vi "Manual Shooter Mode.vi"(10 "Manual Shoot":T1) -> (0 "Shooter Ready?":bool, 1 "Trigger Output":dbl, 2 "Right Output":dbl, 3 "Left Output":dbl, 4 "Angle Motor Out":dbl)   [LabVIEW 2015]
uses:
  Common Code/Manual Shoot.ctl
  Robot Global Data.vi
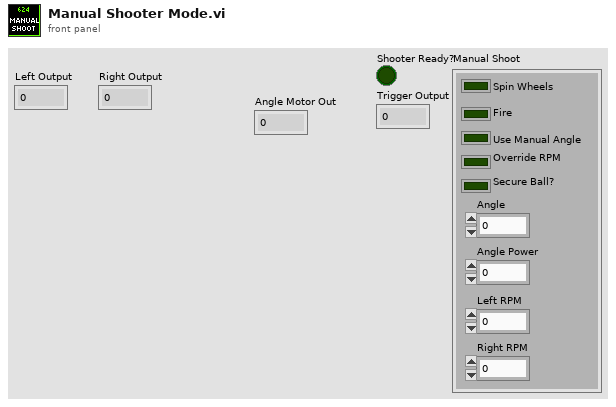
[diagram p1: front panel]
types:
  T1 = typedef "Manual Shoot.ctl" = cluster{"Spin Wheels":bool, "Fire":bool, "Angle":dbl, "Angle Power":dbl, "Use Manual Angle":bool, "Override RPM":bool, "Left RPM":dbl, "Right RPM":dbl, "Secure Ball?":bool}
  T2 = typedef "Dashboard Control Data.ctl" = cluster{"Shooter Presets":T3, "Encoder Control":T5, "Steer PID output":cluster{"output high":dbl, "output low":dbl}, " Steer PID gains":cluster{"proportional gain (Kc)":dbl, "integral time (Ti, min)":dbl, "derivative time (Td, min)":dbl}, "Drivetrain Settings":T6, "Vision Packet":T7, "Dashboard Drivetrain Command":T8, "Info/Command Cluster":T10, "Ball Vision Packet":T11, "Intake Presets":T13, "Intake Encoder Control":T15, "Climb Presets":T16, "Ultrasonic Limit":dbl, "Roll Limit":dbl, "Pitch Limit":dbl, "Goal Output Range":cluster{"output high":dbl, "output low":dbl}}
  T3 = typedef "Shooter Presets.ctl" = cluster{"Batter Shot":T4, "Deep Middle Shot":T4, "Manual Shot":T4, "Left Ticks Per Rotation":dbl, "Right Ticks Per Rotation":dbl, "Low Bar Shot":T4, "Shooter RPM Tolerance":dbl, "IIR Filter Power":dbl, "Trigger Power":dbl, "Fire from Load Delay":i32, "Angle Pot M":dbl, "Angle Pot B":dbl, "Shooter Length":dbl, "String Pot Dist":dbl, "Angle PID gains":cluster{"proportional gain (Kc)":dbl, "integral time (Ti, min)":dbl, "derivative time (Td, min)":dbl}, "Angle Motor Output":cluster{"output high":dbl, "output low":dbl}, "Shooter Angle Tolerance":dbl, "Vision Shoot x^2":dbl, "Vision Shoot x":dbl, "Dist from Axis Cam to Pivot":dbl, "High Goal Center Height":dbl, "Feed Forward Max Accel":dbl, "Feed Forward Kv":dbl, "Backwards Trigger":dbl, "Shot Finish Delay (ms)":dbl, "Angle Max Current":dbl, "Angle Current Trip Time":dbl, "Shooter Intake Angle":dbl, "Vision Shoot c":dbl, "Reset?":bool, "Servo Release Delay":dbl, "Servo Idle Angle":i32, "Servo Hold Angle":i32, "Angle Pot x^2":dbl, "Angle Pot x":dbl, "Angle Pot c":dbl, "Ignore Angle?":bool}
  T4 = typedef "Shot Presets.ctl" = cluster{"Left Wheel RPM":dbl, "Right Wheel RPM":dbl, "Angle":dbl}
  T5 = typedef "Encoder Control.ctl" = cluster{"Right Tick Constant":dbl, "Left Tick Constant":dbl, "Reset?":bool, "Y Dist":cluster{"PID gains":cluster{"proportional gain (Kc)":dbl, "integral time (Ti, min)":dbl, "derivative time (Td, min)":dbl}}, "Y Stop Thresh":dbl, "Y Stop Speed":dbl}
  T6 = typedef "Drivetrain Settings.ctl" = cluster{"Gyro Tolerance":dbl, "Throttle Ramp (ms)":dbl, "Angular rate compensation":bool, "Throttle to Rate Scale":dbl, "Rate compensation gain":dbl, "Kv":dbl, "Ka":dbl, "Feed Forward P":dbl, "Feed Forward D":dbl, "Goal Vision PID gains":cluster{"proportional gain (Kc)":dbl, "integral time (Ti, min)":dbl, "derivative time (Td, min)":dbl}, "Goal Detection Window":dbl}
  T7 = typedef "Goal Vision Packet.ctl" = cluster{"Distance":dbl, "Center X":dbl, "Center Y":dbl, "Found Target?":bool}
  T8 = typedef "Dashboard Drivetrain Command.ctl" = cluster{"Drivetrain Vision":T9}
  T9 = typedef "Drivetrain Vision.ctl" = cluster{"Goal Window":dbl, "Ball Window":dbl}
  T10 = typedef "Ball Tracking Command Cluster.ctl" = cluster{"Distance to Ball":dbl, "Desired Angle":dbl, "Command":enum16{"Turn to Ball", "Turn to Angle", "Get Distance"}, "Pixels from Center":dbl}
  T11 = typedef "Ball Vision Packet.ctl" = cluster{"Ball Detected?":bool, "Distance to Ball":dbl, "Desired Angle":dbl, "Pixels from Center":dbl, "Tracking mode":T12}
  T12 = typedef "Tracking Mode.ctl" = enum16{"Turn to Ball", "Turn to Angle"}
  T13 = typedef "Intake Presets.ctl" = cluster{"Intake Speed":dbl, "Outake Speed":dbl, "Low Height":dbl, "Half Height":dbl, "Full Height":dbl, "Angle Speed":dbl, "Fast Angle":dbl, "Encoder Scale":dbl, "Load Height":dbl, "Output Range":T14, "Rotation Power Max/Min":dbl, "MaxCurrent":dbl, "Intake Trip Time":dbl, "Idle Height":dbl, "Max Height":dbl, "Reset Encoders?":bool, "PID gains":cluster{"proportional gain (Kc)":dbl, "integral time (Ti, min)":dbl, "derivative time (Td, min)":dbl}}
  T14 = typedef "Drivetrain Output Range.ctl" = cluster{"output high":dbl, "output low":dbl}
  T15 = typedef "IntakeEcoderControl.ctl" = cluster{"Arm Tick Constant":dbl, "Reset?":bool, "Y Dist":cluster{"PID gains":cluster{"proportional gain (Kc)":dbl, "integral time (Ti, min)":dbl, "derivative time (Td, min)":dbl}}, "Y Stop Thresh":dbl, "Y Stop Speed":dbl}
  T16 = typedef "Climb Presets.ctl" = cluster{"Pull Power":dbl, "Unpin Power":dbl, "Time to Hold":dbl}
  T17 = typedef "WPI_MotorControlDeviceRef.ctl" = cluster{"DeviceStatus":errorcluster, "Type":T18, "PWM":cluster{"PWM Channel":T19, "DeadBand":T20}, "CAN":cluster{"Device Number":u8, "Control Mode":T21, "Semaphore":T22, "Max Vout":dbl, "TalonSRX Control Mode":T23}, "Invert":bool}
  T18 = typedef "WPI_MotorControlType.ctl" = enum16{"PWM", "CAN", "CANTalonSRX"}
  T19 = typedef "FPGA_DIOPWMChannel.ctl" = enum8{"PWM 0", "PWM 1", "PWM 2", "PWM 3", "PWM 4", "PWM 5", "PWM 6", "PWM 7", "PWM 8", "PWM 9", "PWM MXP 0", "PWM MXP 1", "PWM MXP 2", "PWM MXP 3", "PWM MXP 4", "PWM MXP 5", "PWM MXP 6", "PWM MXP 7", "PWM MXP 8", "PWM MXP 9", "Invalid"}
  T20 = typedef "WPI_PWMDeadband.ctl" = cluster{"Name":string, "maxPositivePwm":i32, "minPositivePwm":i32, "centerPwm":i32, "maxNegativePwm":i32, "minNegativePwm":i32, "angularRange":u16}
  T21 = typedef "WPI_CANJaguar_ControlMode.ctl" = enum8{"Percent VBus", "Current", "Speed", "Position", "Voltage"}
  T22 = typedef "Semaphore RefNum" = refnum<k1>
  T23 = typedef "WPI_CANTalonSRX_APIControlMode.ctl" = enum8{"Percent VBus", "Speed", "Position", "Slave", "Unchanged / Invalid", "Voltage Compensation", "Current", "Motion Profile"}
  T24 = typedef "Intake Status Cluster.ctl" = cluster{"Roller Power":dbl, "Angle Power":dbl, "Intake Mode":T25, "Intake States":T26, "Rollers Active?":bool, "Current Height":dbl, "Target Height":dbl, "Encoder Raw Position":dbl, "Forward Tripped?":bool, "Backward Tripped?":bool, "Override IR?":bool}
  T25 = typedef "Intake Mode.ctl" = enum16{"Safe", "Auto", "Manual"}
  T26 = typedef "Intake States.ctl" = enum16{"Idle", "Set roller speed", "Move to angle"}
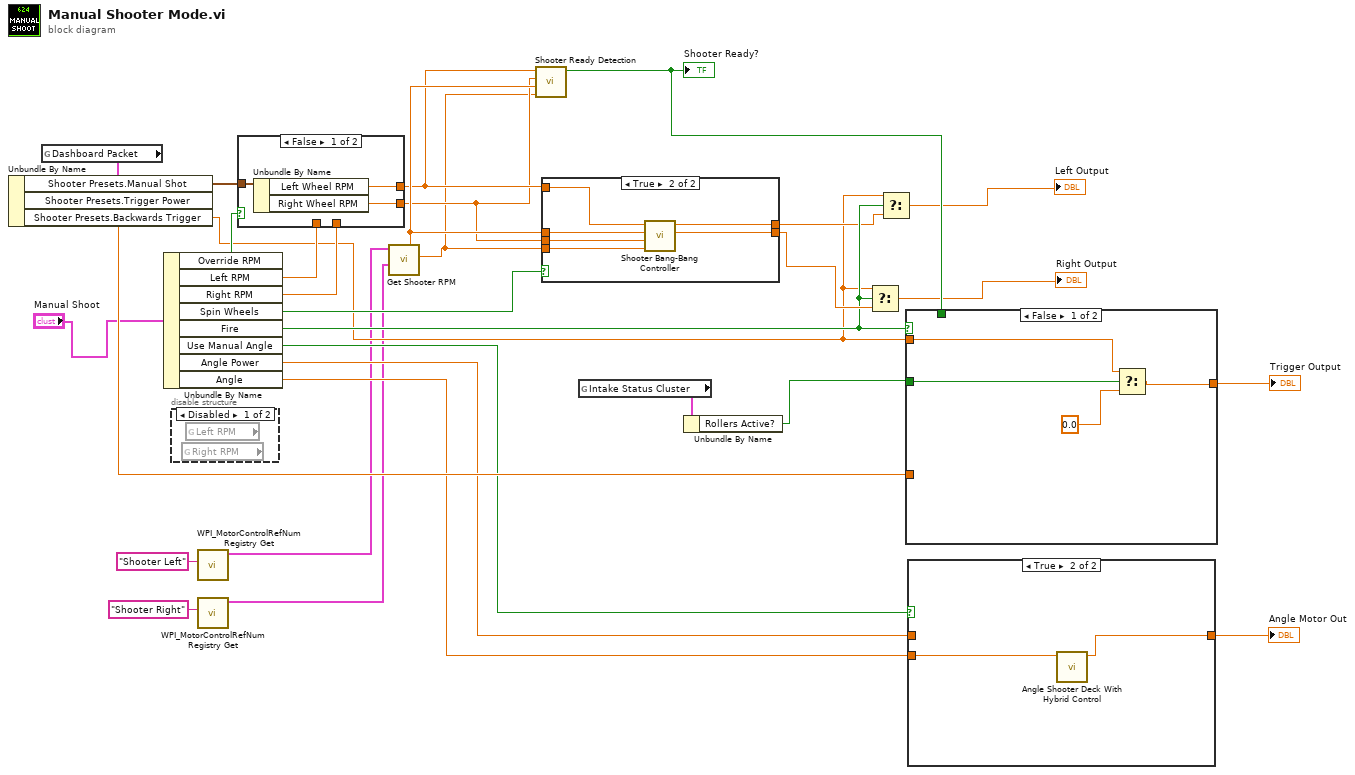
[diagram p0: block diagram]
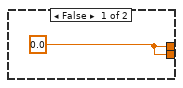
[diagram p6: hidden frame]
diagram:
  n1 = global read "Robot Global Data.vi" "Dashboard Packet"() -> (w30:T2)
  n2 = Unbundle By Name(w30) -> ("Shooter Presets.Manual Shot"=w29:T4, "Shooter Presets.Trigger Power"=w20:dbl, "Shooter Presets.Backwards Trigger"=w8:dbl)
  n3 = Unbundle By Name("Manual Shoot") -> ("Override RPM"=w15:bool, "Left RPM"=w14:dbl, "Right RPM"=w13:dbl, "Spin Wheels"=w28:bool, "Fire"=w10:bool, "Use Manual Angle"=w19:bool, "Angle Power"=w17:dbl, "Angle"=w16:dbl)
  n4 = disable-structure shown="Disabled" {
    frame Disabled {
      n5 = global read "Robot Global Data.vi" "Right RPM"() -> ()  [unwired: 1 out]
      n6 = global read "Robot Global Data.vi" "Left RPM"() -> ()  [unwired: 1 out]
    }
    frame Enabled {
    }
  }
  n7 = call <vilib>:"WPI_MotorControlRefNum Registry Get.vi"("refnum name"="Shooter Left") -> ("MotorControlDevRef"=w3:T17)  [unwired: 9 in, 1 out]
  n8 = call <vilib>:"WPI_MotorControlRefNum Registry Get.vi"("refnum name"="Shooter Right") -> ("MotorControlDevRef"=w1:T17)  [unwired: 9 in, 1 out]
  n9 = case shown="False" w15 {
    tunnel: w29 -> [w33 _]
    tunnel: [w32 w35] -> w26
    tunnel: [w31 w34] -> w25
    tunnel: w14 -> [_ w35]
    tunnel: w13 -> [_ w34]
    frame False {
      n10 = Unbundle By Name(w33) -> ("Left Wheel RPM"=w32:dbl, "Right Wheel RPM"=w31:dbl)
    }
    frame True {
    }
  }
  n11 = call "Get Shooter RPM.vi"("Right Shooter Wheel"=w1, "Left Shooter Wheel"=w3) -> ("Right RPM"=w24:dbl, "Left RPM"=w27:dbl)  [unwired: 7 in, 1 out]
  n12 = call "Shooter Ready Detection.vi"("Right RPM"=w24, "Left RPM"=w27, "Right RPM Target"=w25, "Left RPM Target"=w26) -> ("Shooter Ready?"=w23:bool)  [unwired: 7 in]
  "Shooter Ready?" <- w23
  n13 = case shown="True" w28 {
    tunnel: w26 -> [_ w42]
    tunnel: w25 -> [_ w41]
    tunnel: [w36 w40] -> w9
    tunnel: [w36 w39] -> w12
    tunnel: w27 -> [_ w38]
    tunnel: w24 -> [_ w37]
    frame False {
      w36 = 0.0 ("Left Output Power")
    }
    frame True {
      n14 = call "Shooter Bang-Bang Controller.vi"("Right Current RPM"=w37, "Right Target RPM"=w41, "Left Current RPM"=w38, "Left Target RPM"=w42) -> ("Right Output Power"=w39:dbl, "Left Output Power"=w40:dbl)  [unwired: 6 in]
    }
  }
  n15 = global read "Robot Global Data.vi" "Intake Status Cluster"() -> (w6:T24)
  n16 = Unbundle By Name(w6) -> ("Rollers Active?"=w21:bool)
  n17 = Select(t=w8, s=w10, f=w12) -> (s? t:f=→"Right Output":dbl)
  n18 = Select(t=w8, s=w10, f=w9) -> (s? t:f=→"Left Output":dbl)
  n19 = case shown="False" w10 {
    tunnel: w23 -> [_ _]
    tunnel: [w45 w47] -> w22
    tunnel: w21 -> [w43 _]
    tunnel: w20 -> [_ w47]
    tunnel: w8 -> [w44 _]
    frame False {
      n20 = Select(t=w44, s=w43, f=0.0 ("Trigger Output")) -> (s? t:f=w45:dbl)
    }
    frame True {
      # "Fire when Pressed"
    }
  }
  "Trigger Output" <- w22
  n21 = case shown="True" w19 {
    tunnel: [w48 w49] -> w18
    tunnel: w17 -> [w48 _]
    tunnel: w16 -> [_ w50]
    frame False {
    }
    frame True {
      n22 = call "Angle Shooter Deck With Hybrid Control.vi"("Target Angle"=w50) -> ("Angle Motor Power Out"=w49:dbl)  [unwired: 10 in]
    }
  }
  "Angle Motor Out" <- w18
